vi "MicroPulse - Data Receive.vi"(8 "error in (no error)":errorcluster, 9 "disable [F]":bool, 11 "TCP config":T1={"Connection ID"=refnum, "IP address"="10.1.1.2", "host port"=1067, "OC timeout"=-1, "Read timeout"=0, "Write timeout"=0} {"Write timeout" format="%dms"; "Read timeout" format="%dms"; "OC timeout" format="%dms"}) -> (0 "error out":errorcluster, 1 "total msg length":i32, 2 "data message":string, 3 "TCP config out":T1={"Connection ID"=refnum, "IP address"="10.1.1.2", "host port"=1067, "OC timeout"=-1, "Read timeout"=0, "Write timeout"=0} {"Write timeout" format="%dms"; "Read timeout" format="%dms"; "OC timeout" format="%dms"}, 4 "Rx timeout":bool, 5 "Header Byte":u8 format="%.0x")   [LabVIEW 2026, in "MicroPulse_Driver.lvlib"]
uses:
  MicroPulse_Driver.lvlib
  Public/Data/Datatypes/TCP config.ctl
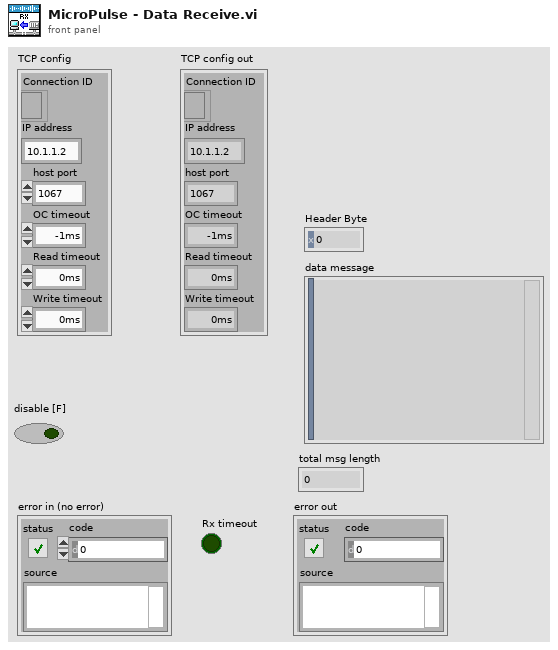
[diagram p1: front panel]
types:
  T1 = typedef "MicroPulse_Driver.lvlib/TCP config.ctl" = cluster{"Connection ID":refnum<k5>, "IP address":string, "host port":u16, "OC timeout":i32, "Read timeout":i32, "Write timeout":i32}
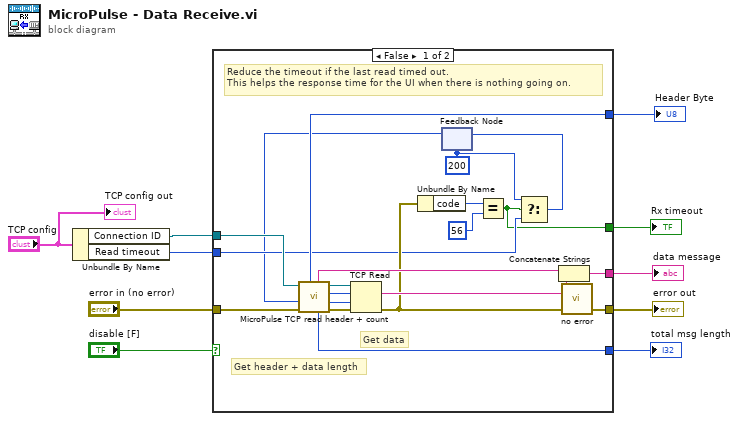
[diagram p0: block diagram]
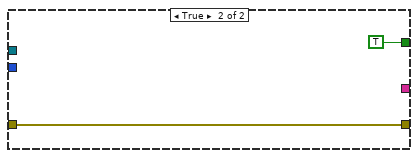
[diagram p2: hidden frame]
diagram:
  n1 = Unbundle By Name("TCP config") -> ("Connection ID"=w3:refnum<k5>, "Read timeout"=w4:i32)
  n2 = case shown="False" "disable [F]" {
    tunnel: [w29 _] -> w8
    tunnel: [w21 w32] -> w9
    tunnel: "error in (no error)" -> [w26 w32]
    tunnel: w4 -> [w13 _]
    tunnel: [w22 _] -> w6
    tunnel: [w11 TRUE ("status")] -> w5
    tunnel: w3 -> [w20 _]
    tunnel: [w19 _] -> w1
    frame False {
      w15 = 200 ("t")
      # "Reduce the timeout if the last read timed out.\nThis helps the response time for the UI when there is nothing going on."
      # "Get header + data length"
      # "Get data"
      n3 = feedback #1(w15) -> (w12:i32)
      n4 = call "MicroPulse TCP read header + count.vi"("error in (no error)"=w26, "TCP timeout"=w12, "connection ID"=w20) -> ("error out"=w27:errorcluster, "TCP timeout"=w23:i32, "bytes to read"=w30:i32, "connection ID out"=w25:refnum<k5>, "total msg length"=w22:i32, "hdr (+count)"=w24:string, "Header Byte"=w19:u8)  [unwired: 2 in]
      n5 = TCP Read(connection ID=w25, bytes to read=w30, error in (no error)=w27, 9:w23) -> (data out=w28:string, error out=w18:errorcluster)  [unwired: 1 in, 1 out]
      n6 = Unbundle By Name(w18) -> ("code"=w17:i32)
      n7 = Equal?(x=w17, y=56) -> (x = y?=w11:bool)
      n8 = Select(t=w15, s=w11, f=w13) -> (s? t:f=w14:i32)
      n9 = feedback-in #1(w14) -> ()
      n10 = Concatenate Strings(w24, w28) -> (w29:string)
      n11 = call "no error.vi"("error in (no error)"=w18) -> ("error out"=w21:errorcluster)  [unwired: 4 in]
    }
    frame True {
    }
  }
  "error out" <- w9
  "data message" <- w8
  "total msg length" <- w6
  "Rx timeout" <- w5
  "Header Byte" <- w1
  "TCP config out" <- "TCP config"
